vi "movimentacao melhor.vi"() -> ()   [LabVIEW 2020]
uses:
  <vilib>/Utility/inputDevices.llb/joystickAcquire.vi
  <vilib>/Utility/inputDevices.llb/closeJoystick.vi
panel:
  out "Acelerando Trás":bool
  out "Acelerando Frente":bool
  out "Motor Direita":bool
  out "Velocidade Motor Direita":dbl(knob) scale=-100.0..100.0 scale format="%#.0p"
  out "Velocidade Motor Esquerda":dbl(knob) scale=-100.0..100.0 scale format="%#.0p"
  out "Motor Esquerda":bool
  out "joystick info":T1(array[cluster])
  out "axis info":T2
  out "button info":T3
  out "direction info":T4
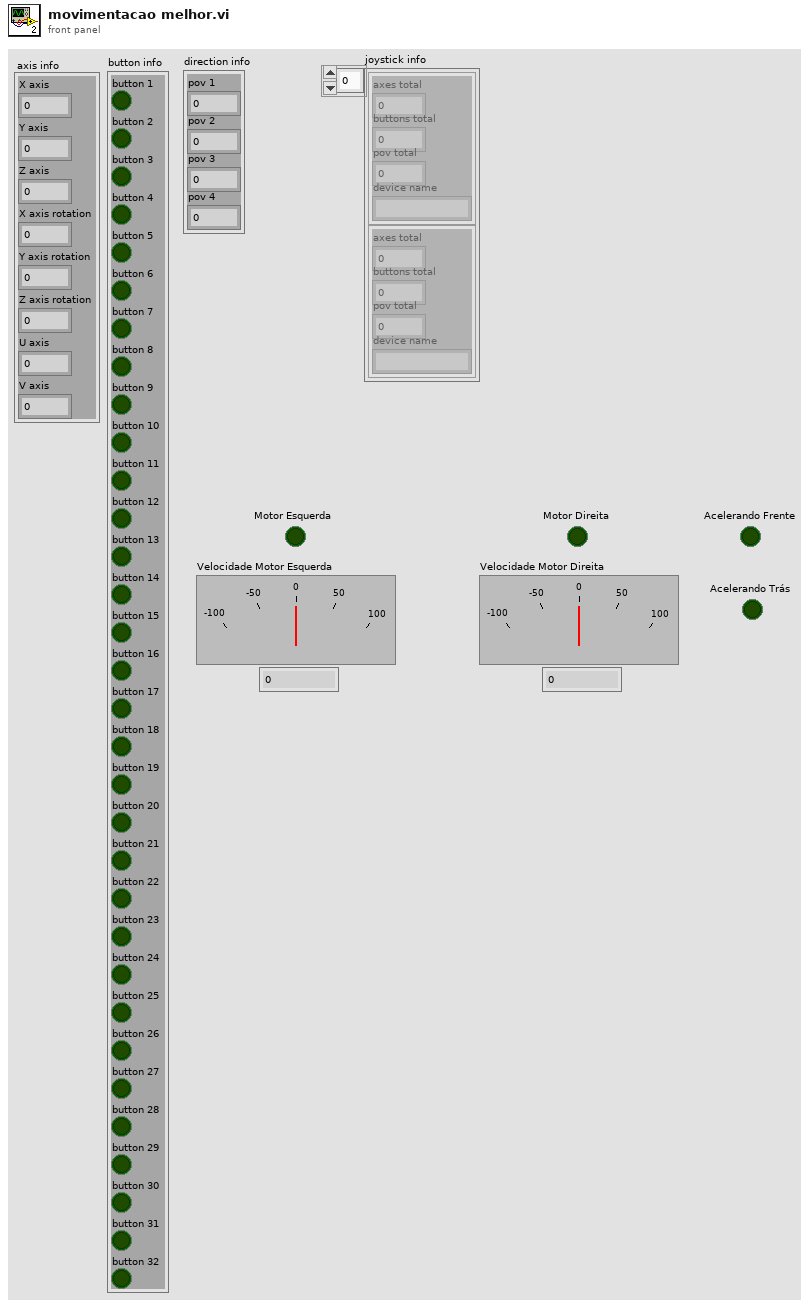
[diagram p1: front panel]
types:
  T1 = cluster{"axes total":u32, "buttons total":u32, "pov total":u32, "device name":string}[]
  T2 = cluster{"X axis":i32, "Y axis":i32, "Z axis":i32, "X axis rotation":i32, "Y axis rotation":i32, "Z axis rotation":i32, "U axis":i32, "V axis":i32}
  T3 = cluster{"button 1":bool, "button 2":bool, "button 3":bool, "button 4":bool, "button 5":bool, "button 6":bool, "button 7":bool, "button 8":bool, "button 9":bool, "button 10":bool, "button 11":bool, "button 12":bool, "button 13":bool, "button 14":bool, "button 15":bool, "button 16":bool, "button 17":bool, "button 18":bool, "button 19":bool, "button 20":bool, "button 21":bool, "button 22":bool, "button 23":bool, "button 24":bool, "button 25":bool, "button 26":bool, "button 27":bool, "button 28":bool, "button 29":bool, "button 30":bool, "button 31":bool, "button 32":bool}
  T4 = cluster{"pov 1":i32, "pov 2":i32, "pov 3":i32, "pov 4":i32}
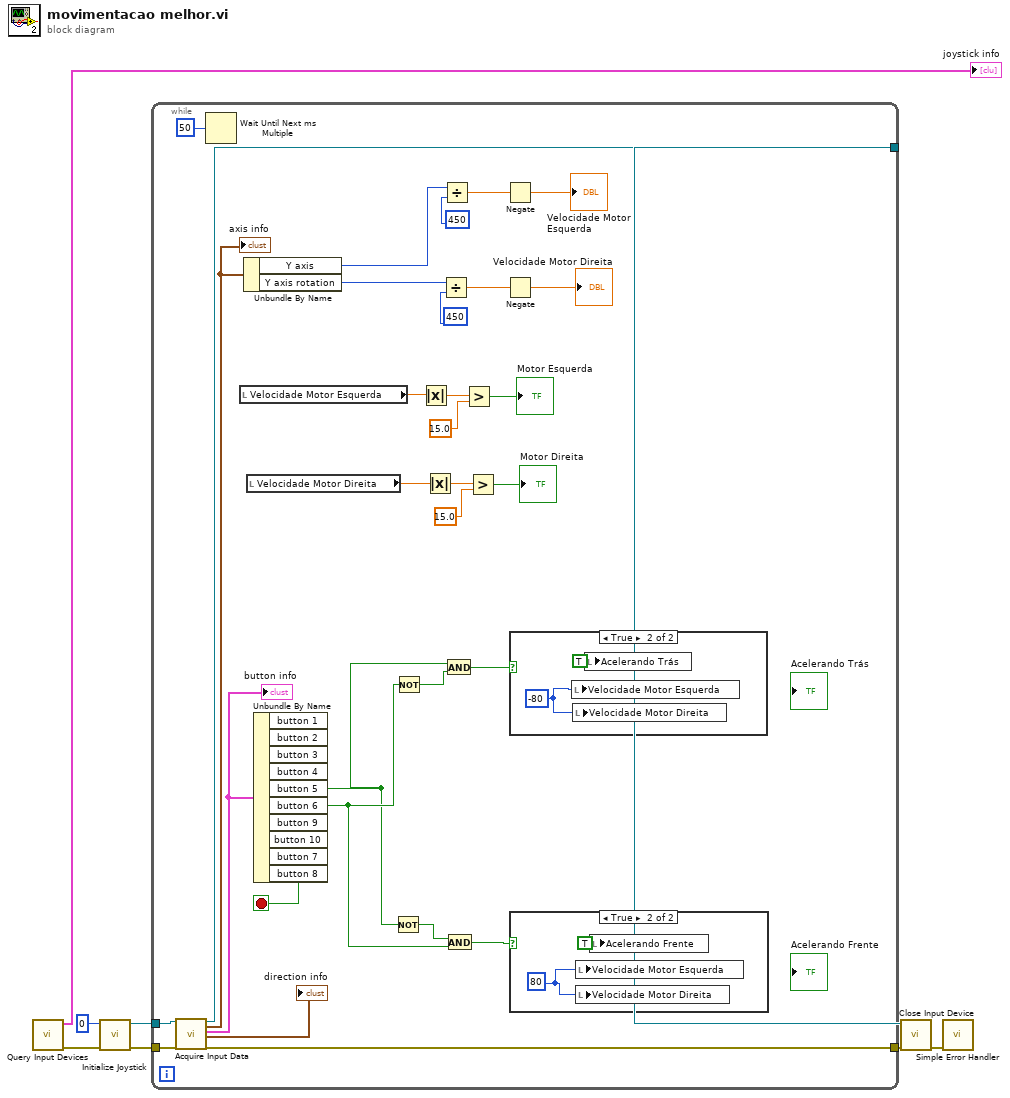
[diagram p0: block diagram]
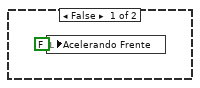
[diagram p2: hidden frame]
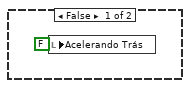
[diagram p3: hidden frame]
diagram:
  n1 = call <vilib>:"Query Input Devices.vi"() -> ("error out"=w2:errorcluster, "joystick info"=→"joystick info":T1)  [unwired: 1 in, 9 out]
  n2 = call <vilib>:"Initialize Joystick.vi"("error in (no error)"=w2, "device index"=0) -> ("error out"=w6:errorcluster, "device ID"=w7:refnum<k1>)  [unwired: 8 out]
  n3 = while {
    tunnel: w7 -> [w39]
    tunnel: w6 -> [w38]
    tunnel: [w37] -> w5
    tunnel: [w34] -> w4
    stop <- w32 stop-if-true
    n4 = call-poly <vilib>:"Acquire Input Data.vi"("device ID"=w39, "error in (no error)"=w38) -> ("device ID"=w37:refnum<k1>, "axis info"=w35:T2, "button info"=w31:T3, "direction info"=→"direction info":T4, "error out"=w34:errorcluster)  [unwired: 13 out]
    "axis info" <- w35
    "button info" <- w31
    n5 = Wait Until Next ms Multiple(millisecond multiple=u32 50) -> ()  [unwired: 1 out]
    n6 = local read "Velocidade Motor Esquerda"() -> (w25:dbl)
    n7 = Unbundle By Name(w35) -> ("Y axis"=w30:i32, "Y axis rotation"=w27:i32)
    n8 = local read "Velocidade Motor Direita"() -> (w20:dbl)
    n9 = Unbundle By Name(w31) -> ("button 5"=w9:bool, "button 6"=w10:bool, "button 7"=w32:bool)  [unwired: 7 out]
    n10 = Not(x=w9) -> (.not. x?=w16:bool)
    n11 = Not(x=w10) -> (.not. x?=w18:bool)
    n12 = Absolute Value(x=w25) -> (abs(x)=w24:dbl)
    n13 = Absolute Value(x=w20) -> (abs(x)=w22:dbl)
    n14 = Divide(x=w27, y=450) -> (x/y=w12:dbl)
    n15 = Divide(x=w30, y=450) -> (x/y=w14:dbl)
    n16 = And(x=w9, y=w18) -> (x .and. y?=w17:bool)
    n17 = And(x=w16, y=w10) -> (x .and. y?=w15:bool)
    n18 = Greater?(x=w24, y=15.0) -> (0:→"Motor Esquerda":bool)
    n19 = Greater?(x=w22, y=15.0) -> (0:→"Motor Direita":bool)
    n20 = Negate(x=w14) -> (-x=→"Velocidade Motor Esquerda":dbl)
    n21 = Negate(x=w12) -> (-x=→"Velocidade Motor Direita":dbl)
    n22 = case shown="True" w17 {
      frame False {
        n23 = local write "Acelerando Trás"(FALSE ("Acelerando Trás")) -> ()
      }
      frame True {
        w45 = -80
        n24 = local write "Velocidade Motor Esquerda"(w45) -> ()
        n25 = local write "Velocidade Motor Direita"(w45) -> ()
        n26 = local write "Acelerando Trás"(TRUE ("Acelerando")) -> ()
      }
    }
    n27 = case shown="True" w15 {
      frame False {
        n28 = local write "Acelerando Frente"(FALSE ("Acelerando Frente")) -> ()
      }
      frame True {
        w42 = 80
        n29 = local write "Velocidade Motor Esquerda"(w42) -> ()
        n30 = local write "Velocidade Motor Direita"(w42) -> ()
        n31 = local write "Acelerando Frente"(TRUE ("Acelerando Frente")) -> ()
      }
    }
  }
  n32 = call-poly <vilib>:"Close Input Device.vi"("error in (no error)"=w4, "device ID"=w5) -> ("error out"=w1:errorcluster)  [unwired: 8 out]
  n33 = call <vilib>:"Simple Error Handler.vi"("error in (no error)"=w1) -> ()  [unwired: 1 in, 8 out]
